vi "Configure Modulation (Amplitude).vi"(0 "VISA resource name":refnum<visa-resource-name>, 1 "Enable Amplitude Modulation (T: Enable)":bool=TRUE, 2 "File Path":string, 5 "Channel (0: Channel 1)":u16(ring) items=["Channel 1", "Channel 2"], 7 "AM Source (0: Internal)":u16(ring) items=["Internal", "External"], 9 "Modulation Waveform (0: Sine)":u16(ring) items=["Sine", "Square", "Triangle", "Ramp", "Down Ramp", "Noise", "User 1", "User 2", "User 3", "User 4", "Edit Memory", "Edit File"], 11 "error in (no error)":errorcluster, 12 "Modulation Frequency (1000 Hz)":dbl=1000.0, 13 "Modulation Depth (0 %)":dbl) -> (4 "VISA resource name out":refnum<visa-resource-name>, 15 "error out":errorcluster)   [LabVIEW 2015, in "Tektronix AFG 3000 Series.lvlib"]
doc: "Configures and enables amplitude modulation (AM). In AM, the amplitude of the carrier is varied by the amplitude of the modulating waveform."
uses:
  Tektronix AFG 3000 Series.lvlib
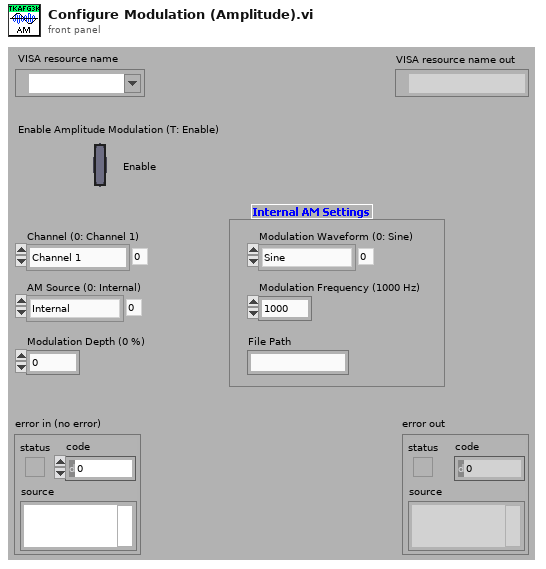
[diagram p1: front panel]
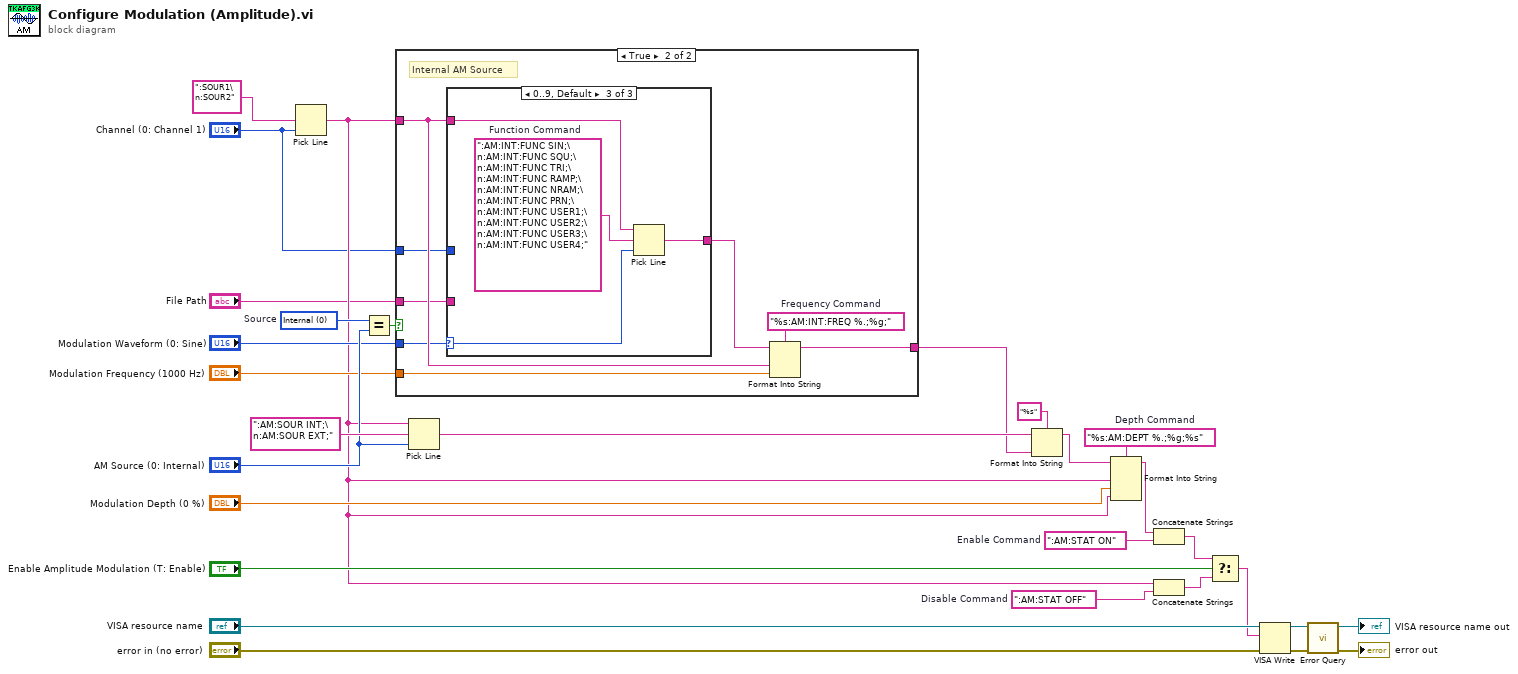
[diagram p0: block diagram]
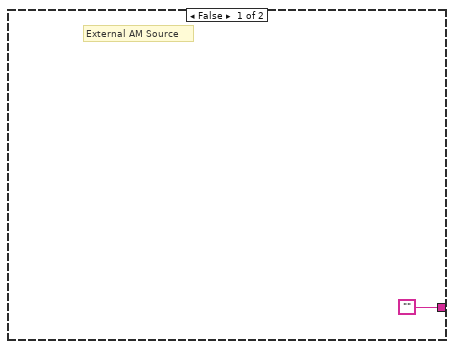
[diagram p2: hidden frame]
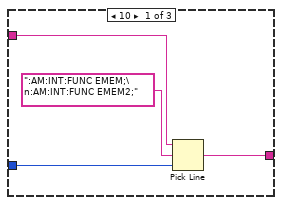
[diagram p3: hidden frame]
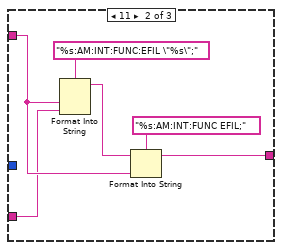
[diagram p4: hidden frame]
diagram:
  w20 = ":AM:STAT ON"  # Enable Command
  w22 = "%s:AM:DEPT %.;%g;%s"  # Depth Command
  w9 = u16 0 items=["Internal", "External"]  # Source
  w16 = ":AM:STAT OFF"  # Disable Command
  n1 = Pick Line(multi-line string=":SOUR1\n:SOUR2" ("string (\"\")"), line index="Channel (0: Channel 1)") -> (output string=w4:string)  [unwired: 1 in]
  n2 = Equal?(x=w9, y="AM Source (0: Internal)") -> (x = y?=w14:bool)
  n3 = case shown="True" w14 {
    tunnel: w4 -> [_ w36]
    tunnel: ["" w37] -> w11
    tunnel: "Modulation Waveform (0: Sine)" -> [_ w34]
    tunnel: "Modulation Frequency (1000 Hz)" -> [_ w35]
    tunnel: "Channel (0: Channel 1)" -> [_ w33]
    tunnel: "File Path" -> [_ w32]
    frame False {
      # "External AM Source"
    }
    frame True {
      w38 = "%s:AM:INT:FREQ %.;%g;"  # Frequency Command
      # "Internal AM Source"
      n4 = case shown="0..9, Default" w34 {
        selector: w34 -> [_ _ w50]
        tunnel: w36 -> [w41 w46 w51]
        tunnel: w33 -> [w40 _ _]
        tunnel: w32 -> [_ w45 _]
        tunnel: [w39 w43 w49] -> w31
        frame 10 {
          n5 = Pick Line(string ("")=w41, multi-line string=":AM:INT:FUNC EMEM;\n:AM:INT:FUNC EMEM2;", line index=w40) -> (output string=w39:string)
        }
        frame 11 {
          n6 = Format Into String(format string="%s:AM:INT:FUNC:EFIL \"%s\";", w46, w45) -> (resulting string=w48:string)  [unwired: 2 in, 1 out]
          n7 = Format Into String(format string="%s:AM:INT:FUNC EFIL;", initial string=w48, w46) -> (resulting string=w43:string)  [unwired: 1 in, 1 out]
        }
        frame 0..9, Default {
          w52 = ":AM:INT:FUNC SIN;\n:AM:INT:FUNC SQU;\n:AM:INT:FUNC TRI;\n:AM:INT:FUNC RAMP;\n:AM:INT:FUNC NRAM;\n:AM:INT:FUNC PRN;\n:AM:INT:FUNC USER1;\n:AM:INT:FUNC USER2;\n:AM:INT:FUNC USER3;\n:AM:INT:FUNC USER4;"  # Function Command
          n8 = Pick Line(string ("")=w51, multi-line string=w52, line index=w50) -> (output string=w49:string)
        }
      }
      n9 = Format Into String(format string=w38, initial string=w31, w36, w35) -> (resulting string=w37:string)  [unwired: 1 in, 1 out]
    }
  }
  n10 = Pick Line(string ("")=w4, multi-line string=":AM:SOUR INT;\n:AM:SOUR EXT;" ("Source Command"), line index="AM Source (0: Internal)") -> (output string=w12:string)
  n11 = Format Into String(format string="%s", initial string=w12, w11) -> (resulting string=w10:string)  [unwired: 1 in, 1 out]
  n12 = Format Into String(format string=w22, initial string=w10, w4, "Modulation Depth (0 %)", w4) -> (resulting string=w21:string)  [unwired: 1 in, 1 out]
  n13 = Concatenate Strings(w21, w20) -> (w18:string)
  n14 = Concatenate Strings(w4, w16) -> (w15:string)
  n15 = Select(t=w18, s="Enable Amplitude Modulation (T: Enable)", f=w15) -> (s? t:f=w19:string)
  n16 = VISA Write(VISA resource name="VISA resource name", write buffer=w19, error in (no error)="error in (no error)") -> (VISA resource name out=w25:refnum<visa-resource-name>, error out=w24:errorcluster)  [unwired: 1 out]
  n17 = call "Error Query.vi"("error in (no error)"=w24, "VISA resource name"=w25) -> ("error out"=→"error out":errorcluster, "VISA resource name out"=→"VISA resource name out":refnum<visa-resource-name>)  [unwired: 6 in, 2 out]
